vi "Process columns.vi"(8 "Dialate":bool, 9 "WaveformGraph in":refnum<vi>, 10 "Lines":i32, 11 "Image Out":T1) -> (1 "Pixels (U16)":u16[][](array[numeric]), 2 "Filtered X":dbl[][](array[numeric]), 3 "Refnum out":T1, 5 "Points":cluster{cluster{dbl, dbl}, cluster{dbl, dbl}}[](array[cluster]))   [LabVIEW 2017]
uses:
  <vilib>/vision/Image Controls.llb/IMAQ Image.ctl
  <vilib>/vision/NI_Vision_Development_Module.lvlib
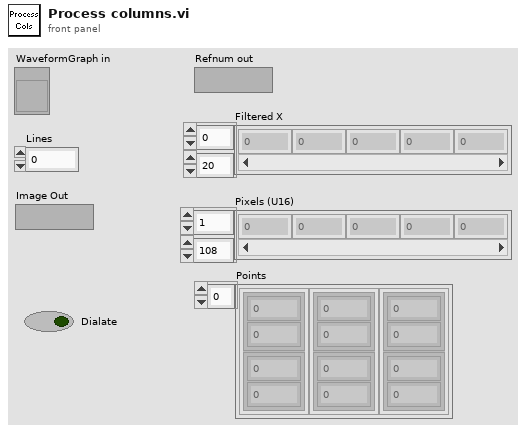
[diagram p1: front panel]
types:
  T1 = typedef "IMAQ Image.ctl" = refnum<image>
  T2 = enum32{"AutoM", "Close", "Dilate", "Erode", "Gradient", "Gradient in", "Gradient out", "HitMiss", "Open", "PClose", "POpen", "Thick", "Thin"}
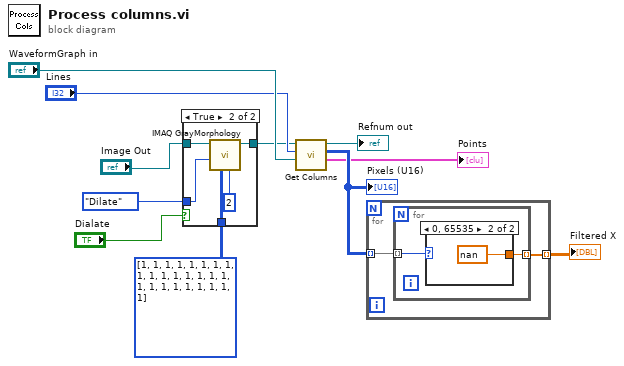
[diagram p0: block diagram]
diagram:
  n1 = case shown="True" "Dialate" {
    tunnel: T2."Dilate" ("Operation") -> [_ w16]
    tunnel: [w12 w15] -> w8
    tunnel: "Image Out" -> [w12 w14]
    tunnel: i32[][] [[1, 1, 1, 1, 1], [1, 1, 1, 1, 1], [1, 1, 1, 1, 1], [1, 1, 1, 1, 1], [1, 1, 1, 1, 1]] ("Structuring Element") -> [_ w13]
    frame False {
    }
    frame True {
      n2 = call "IMAQ GrayMorphology"("Number of iterations (1)"=2, "Structuring Element"=w13, "Operation"=w16, "Image Src"=w14) -> ("Image Dst Out"=w15:T1)  [unwired: 6 in, 1 out]
    }
  }
  n3 = call "Get Columns.vi"("Graph ref"="WaveformGraph in", "Lines"="Lines", "Refnum in"=w8) -> ("Points"=→"Points":cluster{cluster{dbl, dbl}, cluster{dbl, dbl}}[], "Pixels (U16)"=w4:u16[][], "Refnum in 2"=→"Refnum out":T1)  [unwired: 6 in]
  "Pixels (U16)" <- w4
  n4 = for {
    tunnel: w4 -> [w19] mode=indexing
    tunnel: [w18] -> w3 mode=indexing
    n5 = for {
      tunnel: w19 -> [w21] mode=indexing
      tunnel: [w20] -> w18 mode=indexing
      n6 = case shown="0, 65535" w21 {
        selector: w21 -> [w22 _]
        tunnel: [w22 nan] -> w20
        frame Default {
        }
        frame 0, 65535 {
        }
      }
    }
  }
  "Filtered X" <- w3
